vi "TryUpdateGyroSBIT.vi"   [LabVIEW 2016]
uses:
  <vilib>/Platform/TimedLoop/XDataNode/timing_clust.ctl
  <vilib>/Platform/TimedLoop/XDataNode/nitl_modes.ctl
  <vilib>/Platform/TimedLoop/XDataNode/wakeup.ctl
  Telemetry/TelemetryDataTypes.ctl
  Telemetry/TelemetryUpdateModes.ctl
  Telemetry/TelemetryFields.ctl
  <vilib>/rvi/Emulation/niFpgaEmulationIsFPGAContextNoSignature.vi
  <vilib>/rvi/Emulation/niFpgaSctlEmulationGetInTimedLoop.vi
  <vilib>/rvi/errors/niFpgaSetErrorForExecOnDevCompSimple.vi
  <vilib>/rvi/eio/common/nirviEmuReportErrorAndStop.vi
  <vilib>/rvi/DataTransferAndStorage/Container/Common/niFpgaContainerGetUniqueNameForEmu.vi
  <vilib>/rvi/FIFO/Fifo_Resource/nirvififoEmulationSetSize.vi
  <vilib>/rvi/FIFO/Fifo_Resource/nirviFifoEmulationQueueMgr.vi
  <instcachedir>/0/nirviFifoEmulationQueueMgr_E5CAEC123FF24DC58D834DCA3CDAA9B5.lvgen/nirviFifoEmulationQueueMgr_E5CAEC123FF24DC58D834DCA3CDAA9B5_040.vi
  <vilib>/Utility/error.llb/Clear Errors.vi
  <vilib>/rvi/FIFO/Fifo_Resource/nirvififoEmulationCreateLock.vi
  <vilib>/rvi/Emulation/niFpgaProcessEmulError.vi
  <vilib>/rvi/FIFO/Fifo_Resource/nirvififoEmulationObtainLock.vi
  <vilib>/rvi/FIFO/Fifo_Resource/nirvififoEmulationReleaseLock.vi
  <vilib>/rvi/occurrence/nirviWaitOnOccurrenceBase.vi
  <vilib>/rvi/errors/nirviReportUnexpectedCaseInternalError.vi
  <vilib>/rvi/errors/nirviReportUnexpectedCaseInternalError (U32).vi
  <vilib>/rvi/Emulation/niFpgaEmulationReportErrorSimple.vi
  <vilib>/rvi/Emulation/niFpgaGetClockAttributes.vi
  <vilib>/rvi/Emulation/niFpgaCriticalErrorInLSC.vi
  <instcachedir>/0/nirviFifoEmulationQueueMgr_E5CAEC123FF24DC58D834DCA3CDAA9B5.lvgen/nirviFifoEmulationQueueMgr_E5CAEC123FF24DC58D834DCA3CDAA9B5_038.vi
  <vilib>/rvi/FIFO/Fifo_Resource/nirvififoEmulationDetermineInputValidOut.vi
  <vilib>/rvi/Memory/Memory_Emulation/niFpgaMemoryEmulationCacheClearOnFirstRun.vi
  <vilib>/rvi/Memory/Memory_Emulation/nirvimemoryEmulationManagerCache_MakeExclusive.vi
  <vilib>/rvi/Memory/Memory_Emulation/niFpgaMemoryEmulationValidateCache.vi
  <vilib>/rvi/Memory/Memory_Emulation/nirvimemoryEmulationManagerCache_InsertValue.vi
  <vilib>/rvi/Memory/Memory_Emulation/nirvimemoryEmulationManagerCache_ReleaseExclusive.vi
  <vilib>/rvi/Memory/Memory_Emulation/nirvimemoryEmulationManagerCache_GetValue.vi
  <vilib>/rvi/Memory/Memory_Emulation/nirvimemoryEmulationManagerCache_SetValue.vi
  <instcachedir>/0/nirviFifoEmulationQueueMgr_E5CAEC123FF24DC58D834DCA3CDAA9B5.lvgen/nirviFifoEmulationQueueMgr_E5CAEC123FF24DC58D834DCA3CDAA9B5_004.vi
  <vilib>/rvi/DataTransferAndStorage/Container/XNode/niFpgaContainer.xnode
  <vilib>/rvi/FIFO/Fifo_Resource/nirvififoEmulationRead.vi
  <vilib>/Platform/TimedLoop/XDataNode/XDataNode.xnode
  <vilib>/rvi/FIFO/Fifo_Resource/nirvififoEmulationWrite.vi
  <vilib>/rvi/DataTransferAndStorage/Register/Emulation/niFpgaRegisterEmulation.vi
  <vilib>/Platform/TimedLoop/XDataNode/XDNodeRunTimeDep.lvlib
types:
  T1 = cluster{"Timestamp":u64, "TxBytes":u64, "RxBytes":u64, "TxFrames":u64, "RxFrames":u64, "BIT0":u8, "BIT1":u8, "BIT2":u8, "BIT3":u8, "BIT4":u8, "BIT5":u8}
  T2 = typedef "TelemetryFields.ctl" = enum16{"None", "InclinometerTxBytes", "InclinometerRxBytes", "InclinometerTxFrames", "InclinometerRxFrames", "InclinometerErrorTimestamp", "InclinometerErrorCode", "InclinometerSampleTimestamp", "InclinometerRawAngle", "InclinometerZenithAngle", "DisplacementTxBytes", "DisplacementRxBytes", "DisplacementTxFrames", "DisplacementRxFrames", "DisplacementErrorTimestamp", "DisplacementErrorCode", "DisplacementSampleTimestamp", "DisplacementRaw1", "DisplacementRaw2", "DisplacementRaw3", "DisplacementRaw4", "DisplacementRaw5", "DisplacementRaw6", "DisplacementRaw7", "DisplacementRaw8", "DisplacementEng1", "DisplacementEng2", "DisplacementEng3", "DisplacementEng4", "DisplacementEng5", "DisplacementEng6", "DisplacementEng7", "DisplacementEng8", "DisplacementPositionX", "DisplacementPositionY", "DisplacementPositionZ", "DisplacementRotationX", "DisplacementRotationY", "DisplacementRotationZ", "AccelerometerSampleCount", "AccelerometerSampleTimestamp", "AccelerometerRaw1", "AccelerometerRaw2", "AccelerometerRaw3", "AccelerometerRaw4", "AccelerometerRaw5", "AccelerometerRaw6", "AccelerometerRaw7", "AccelerometerRaw8", "AccelerometerEng1", "AccelerometerEng2", "AccelerometerEng3", "AccelerometerEng4", "AccelerometerEng5", "AccelerometerEng6", "AccelerometerEng7", "AccelerometerEng8", "AngularAccelerationX", "AngularAccelerationY", "AngularAccelerationZ", "GyroTxBytes", "GyroRxBytes", "GyroTxFrames", "GyroRxFrames", "GyroErrorTimestamp", "GyroErrorCode", "GyroSampleTimestamp", "AngularVelocityX", "AngularVelocityY", "AngularVelocityZ", "GyroStatus", "GyroSequenceNumber", "GyroTemperature", "GyroBITTimestamp", "GyroBIT0", "GyroBIT1", "GyroBIT2", "GyroBIT3", "GyroBIT4", "GyroBIT5", "GyroBIT6", "GyroBIT7"}
  T3 = typedef "TelemetryUpdateModes.ctl" = enum8{"=", "+", "-", "|"}
  T4 = typedef "TelemetryDataTypes.ctl" = enum8{"U8", "U16", "U32", "U64", "I8", "I16", "I32", "I64", "SGL"}
  T5 = typedef "XDNodeRunTimeDep.lvlib/timing_clust.ctl" = cluster{"Expected End [f-1]":u64, "Actual End [f-1]":u64, "Finished Late? [f-1]":bool, "Expected End [i-1]":u64, "Actual End [i-1]":u64, "Finished Late? [i-1]":bool, "Expected Start [i]":u64, "Actual Start [i]":u64, "Expected Start [f]":u64, "Actual Start [f]":u64, "Source Name":string, "Structure Name":string, "Period":i64, "Deadline":i64, "Offset":i64, "Start":i64, "Priority":i32, "Timeout":i32, "Mode":T6, "Wakeup Reason":T7, "Error":errorcluster, "Source Type":string, "Secondary Source Type":string, "Global End Time":u64, "Global Start Time":u64, "Frame Duration":u64, "Iteration Duration":u64, "Assigned CPU":i32, "I/O Scan Engine Mode":u32}
  T6 = typedef "XDNodeRunTimeDep.lvlib/nitl_modes.ctl" = enum32{"No Change", "Process missed periods, maintain original phase", "Discard missed periods, maintain original phase", "Process missed periods, ignore original phase", "Discard missed periods, ignore original phase"}
  T7 = typedef "XDNodeRunTimeDep.lvlib/wakeup.ctl" = enum32{"Normal", "Aborted", "Asynchronous wakeup", "Timing source error", "Timed loop error", "Timeout"}
  T8 = typedef "TelemetryUpdateData.ctl" = cluster{"DataType":T4, "Mode":T3, "Field":T2, "Data":u64}
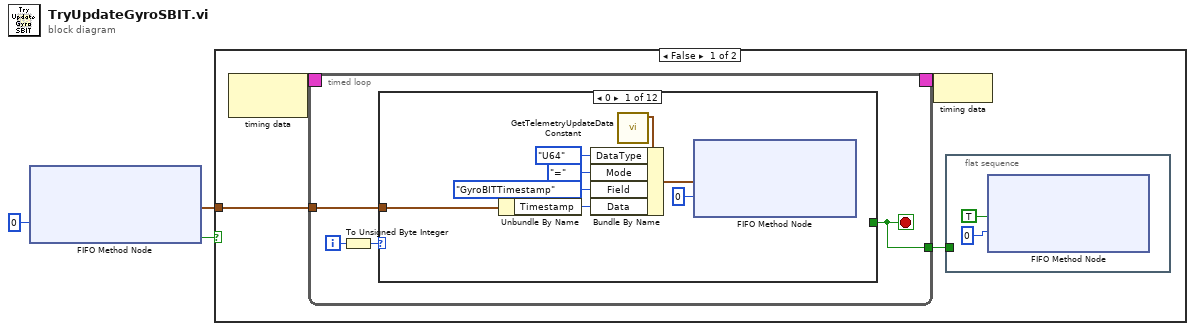
[diagram p0: block diagram]
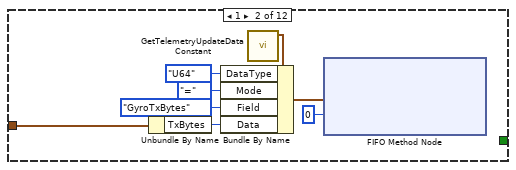
[diagram p2: hidden frame]
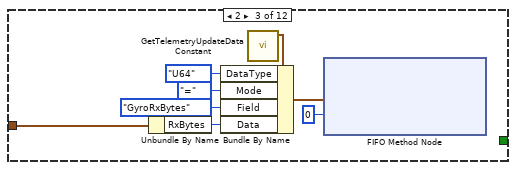
[diagram p3: hidden frame]
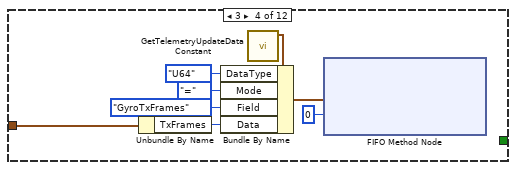
[diagram p4: hidden frame]
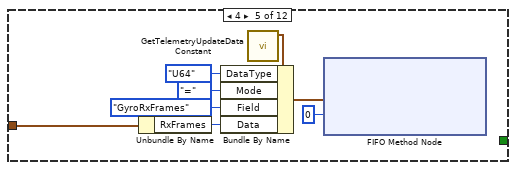
[diagram p5: hidden frame]
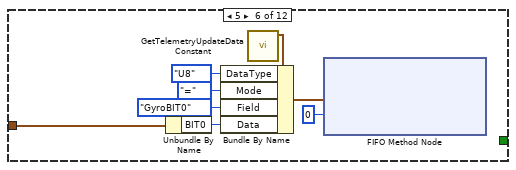
[diagram p6: hidden frame]
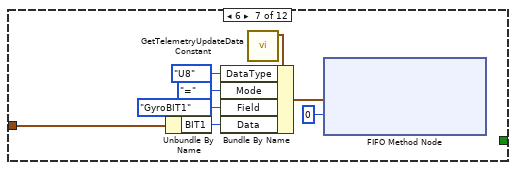
[diagram p7: hidden frame]
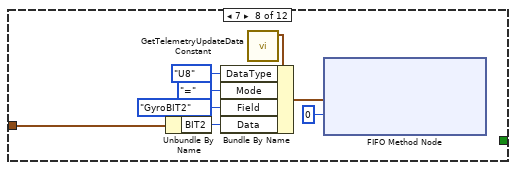
[diagram p8: hidden frame]
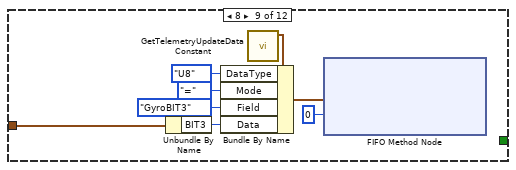
[diagram p9: hidden frame]
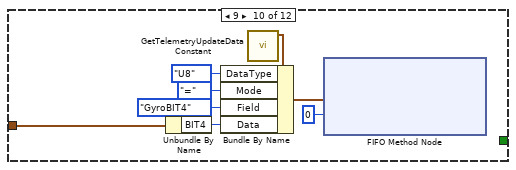
[diagram p10: hidden frame]
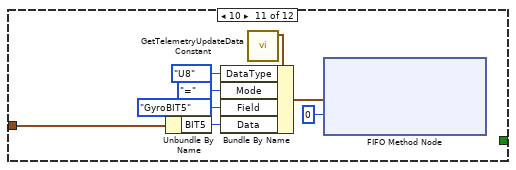
[diagram p11: hidden frame]
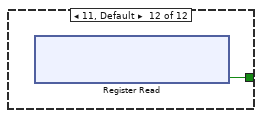
[diagram p12: hidden frame]
diagram:
  n1 = xnode ("FIFO Method Node")("Timeout"=0) -> ("Element"=w1:T1, "Timed Out?"=w2:bool)  [unwired: 1 in, 1 out]
  n2 = case shown="False" w2 {
    tunnel: w1 -> [w7 _]
    frame False {
      n3 = node-c288() -> (w6:T5)  [unwired: 1 in]
      n4 = timed-loop {
        tunnel: w7 -> [w11]
        timing: w6 -> [_]
        timing-out: [_] -> w5
        tunnel: [w10] -> w4
        i -> [w9]
        stop <- w10 stop-if-true
        n5 = To Unsigned Byte Integer(number=w9) -> (unsigned 8bit integer=w8:u8)
        n6 = case shown="0" w8 {
          tunnel: w11 -> [w12 w20 w28 w36 w44 w52 w60 w68 w76 w84 w92 _]
          tunnel: [_ _ _ _ _ _ _ _ _ _ _ w100] -> w10
          frame 0 {
            n7 = Unbundle By Name(w12) -> ("Timestamp"=w18:u64)
            n8 = call "GetTelemetryUpdateDataConstant.vi"() -> ("TelemetryUpdateData"=w17:T8)  [unwired: 11 in]
            n9 = Bundle By Name(cluster=w17, "DataType"=TelemetryDataTypes."U64", "Mode"=TelemetryUpdateModes."=", "Field"=TelemetryFields."GyroBITTimestamp" ("TelemetryFields"), "Data"=w18) -> (w14:T8)
            n10 = xnode ("FIFO Method Node")("Element"=w14, "Timeout"=0) -> ()  [unwired: 1 in, 2 out]
          }
          frame 1 {
            n11 = Unbundle By Name(w20) -> ("TxBytes"=w21:u64)
            n12 = call "GetTelemetryUpdateDataConstant.vi"() -> ("TelemetryUpdateData"=w22:T8)  [unwired: 11 in]
            n13 = Bundle By Name(cluster=w22, "DataType"=TelemetryDataTypes."U64", "Mode"=TelemetryUpdateModes."=", "Field"=TelemetryFields."GyroTxBytes", "Data"=w21) -> (w26:T8)
            n14 = xnode ("FIFO Method Node")("Element"=w26, "Timeout"=0) -> ()  [unwired: 1 in, 2 out]
          }
          frame 2 {
            n15 = Unbundle By Name(w28) -> ("RxBytes"=w35:u64)
            n16 = call "GetTelemetryUpdateDataConstant.vi"() -> ("TelemetryUpdateData"=w34:T8)  [unwired: 11 in]
            n17 = Bundle By Name(cluster=w34, "DataType"=TelemetryDataTypes."U64", "Mode"=TelemetryUpdateModes."=", "Field"=TelemetryFields."GyroRxBytes", "Data"=w35) -> (w30:T8)
            n18 = xnode ("FIFO Method Node")("Element"=w30, "Timeout"=0) -> ()  [unwired: 1 in, 2 out]
          }
          frame 3 {
            n19 = Unbundle By Name(w36) -> ("TxFrames"=w37:u64)
            n20 = call "GetTelemetryUpdateDataConstant.vi"() -> ("TelemetryUpdateData"=w38:T8)  [unwired: 11 in]
            n21 = Bundle By Name(cluster=w38, "DataType"=TelemetryDataTypes."U64", "Mode"=TelemetryUpdateModes."=", "Field"=TelemetryFields."GyroTxFrames", "Data"=w37) -> (w42:T8)
            n22 = xnode ("FIFO Method Node")("Element"=w42, "Timeout"=0) -> ()  [unwired: 1 in, 2 out]
          }
          frame 4 {
            n23 = Unbundle By Name(w44) -> ("RxFrames"=w51:u64)
            n24 = call "GetTelemetryUpdateDataConstant.vi"() -> ("TelemetryUpdateData"=w50:T8)  [unwired: 11 in]
            n25 = Bundle By Name(cluster=w50, "DataType"=TelemetryDataTypes."U64", "Mode"=TelemetryUpdateModes."=", "Field"=TelemetryFields."GyroRxFrames", "Data"=w51) -> (w46:T8)
            n26 = xnode ("FIFO Method Node")("Element"=w46, "Timeout"=0) -> ()  [unwired: 1 in, 2 out]
          }
          frame 5 {
            n27 = Unbundle By Name(w52) -> ("BIT0"=w53:u8)
            n28 = call "GetTelemetryUpdateDataConstant.vi"() -> ("TelemetryUpdateData"=w54:T8)  [unwired: 11 in]
            n29 = Bundle By Name(cluster=w54, "DataType"=TelemetryDataTypes."U8", "Mode"=TelemetryUpdateModes."=", "Field"=TelemetryFields."GyroBIT0" ("TelemetryFields"), "Data"=w53) -> (w57:T8)
            n30 = xnode ("FIFO Method Node")("Element"=w57, "Timeout"=0) -> ()  [unwired: 1 in, 2 out]
          }
          frame 6 {
            n31 = Unbundle By Name(w60) -> ("BIT1"=w61:u8)
            n32 = call "GetTelemetryUpdateDataConstant.vi"() -> ("TelemetryUpdateData"=w62:T8)  [unwired: 11 in]
            n33 = Bundle By Name(cluster=w62, "DataType"=TelemetryDataTypes."U8", "Mode"=TelemetryUpdateModes."=", "Field"=TelemetryFields."GyroBIT1" ("TelemetryFields"), "Data"=w61) -> (w65:T8)
            n34 = xnode ("FIFO Method Node")("Element"=w65, "Timeout"=0) -> ()  [unwired: 1 in, 2 out]
          }
          frame 7 {
            n35 = Unbundle By Name(w68) -> ("BIT2"=w69:u8)
            n36 = call "GetTelemetryUpdateDataConstant.vi"() -> ("TelemetryUpdateData"=w70:T8)  [unwired: 11 in]
            n37 = Bundle By Name(cluster=w70, "DataType"=TelemetryDataTypes."U8", "Mode"=TelemetryUpdateModes."=", "Field"=TelemetryFields."GyroBIT2" ("TelemetryFields"), "Data"=w69) -> (w73:T8)
            n38 = xnode ("FIFO Method Node")("Element"=w73, "Timeout"=0) -> ()  [unwired: 1 in, 2 out]
          }
          frame 8 {
            n39 = Unbundle By Name(w76) -> ("BIT3"=w77:u8)
            n40 = call "GetTelemetryUpdateDataConstant.vi"() -> ("TelemetryUpdateData"=w78:T8)  [unwired: 11 in]
            n41 = Bundle By Name(cluster=w78, "DataType"=TelemetryDataTypes."U8", "Mode"=TelemetryUpdateModes."=", "Field"=TelemetryFields."GyroBIT3" ("TelemetryFields"), "Data"=w77) -> (w81:T8)
            n42 = xnode ("FIFO Method Node")("Element"=w81, "Timeout"=0) -> ()  [unwired: 1 in, 2 out]
          }
          frame 9 {
            n43 = Unbundle By Name(w84) -> ("BIT4"=w85:u8)
            n44 = call "GetTelemetryUpdateDataConstant.vi"() -> ("TelemetryUpdateData"=w86:T8)  [unwired: 11 in]
            n45 = Bundle By Name(cluster=w86, "DataType"=TelemetryDataTypes."U8", "Mode"=TelemetryUpdateModes."=", "Field"=TelemetryFields."GyroBIT4" ("TelemetryFields"), "Data"=w85) -> (w89:T8)
            n46 = xnode ("FIFO Method Node")("Element"=w89, "Timeout"=0) -> ()  [unwired: 1 in, 2 out]
          }
          frame 10 {
            n47 = Unbundle By Name(w92) -> ("BIT5"=w93:u8)
            n48 = call "GetTelemetryUpdateDataConstant.vi"() -> ("TelemetryUpdateData"=w94:T8)  [unwired: 11 in]
            n49 = Bundle By Name(cluster=w94, "DataType"=TelemetryDataTypes."U8", "Mode"=TelemetryUpdateModes."=", "Field"=TelemetryFields."GyroBIT5" ("TelemetryFields"), "Data"=w93) -> (w97:T8)
            n50 = xnode ("FIFO Method Node")("Element"=w97, "Timeout"=0) -> ()  [unwired: 1 in, 2 out]
          }
          frame 11, Default {
            n51 = xnode ("Register Read")() -> ("Data"=w100:bool)  [unwired: 1 in, 1 out]
          }
        }
      }
      n52 = node-c288(w5) -> ()
      n53 = flat-sequence {
        tunnel: w4 -> [_]
        frame #0 {
          n54 = xnode ("FIFO Method Node")("Element"=TRUE, "Timeout"=0) -> ()  [unwired: 1 in, 2 out]
        }
      }
    }
    frame True {
    }
  }
